vi "convert freq power interp data.vi"(11 "file path (dialog if empty)":path=path "C:/Users/Ouyang Group/Documents/Data/8-5-16/wavetek power calibration double sweep -4dbm interp 3") -> (3 "Array":cluster{dbl, dbl}[](array[cluster]))   [LabVIEW 2012]
uses:
  <vilib>/Utility/file.llb/Read From Spreadsheet File (DBL).vi
panel:
  out "all rows":dbl[][](array[numeric]) format="%0.3f"
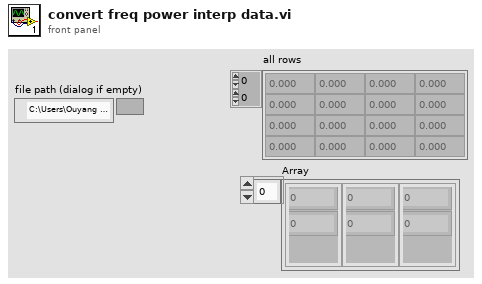
[diagram p1: front panel]
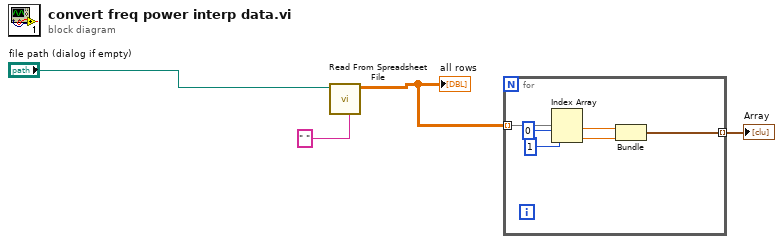
[diagram p0: block diagram]
diagram:
  n1 = call-poly <vilib>:"Read From Spreadsheet File.vi"("delimiter (\\t)"=" " ("delimiter (\\t)"), "file path (dialog if empty)"="file path (dialog if empty)") -> ("all rows"=w3:dbl[][])  [unwired: 5 in, 4 out]
  "all rows" <- w3
  n2 = for {
    tunnel: w3 -> [w10] mode=indexing
    tunnel: [w7] -> w2 mode=indexing
    n3 = Index Array(array=w10, index #1=0 ("index"), index #2=1 ("index")) -> (element #1=w5:dbl, element #2=w6:dbl)
    n4 = Bundle(w5, w6) -> (w7:cluster{dbl, dbl})  [unwired: 1 in]
  }
  "Array" <- w2
